vi "TemperatureToResistance.vi"(1 "Temperature / C":dbl=25.0, 2 "Bridge settings":T1) -> (0 "Resistance / Ohms":dbl=6247.958889803574 format="%0.2f")   [LabVIEW 2015]
uses:
  controls/BridgeSettings.ctl
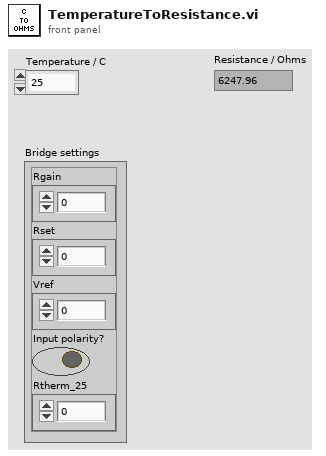
[diagram p1: front panel]
types:
  T1 = typedef "BridgeSettings.ctl" = cluster{"Rgain":dbl, "Rset":dbl, "Vref":dbl, "Input polarity?":bool, "Rtherm_25":dbl}
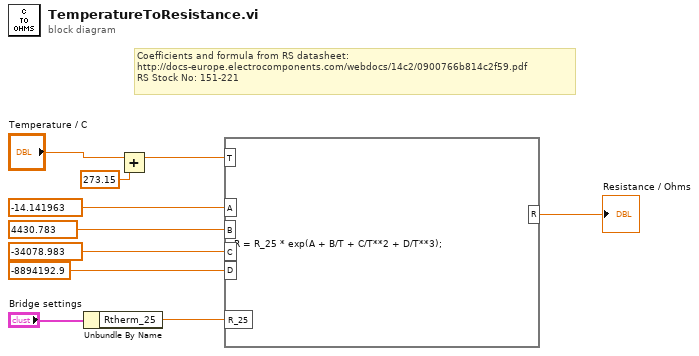
[diagram p0: block diagram]
diagram:
  # "Coefficients and formula from RS datasheet:\nhttp://docs-europe.electrocomponents.com/webdocs/14c2/0900766b814c2f59.pdf\nRS Stock No: 151-221"
  n1 = Unbundle By Name("Bridge settings") -> ("Rtherm_25"=w1:dbl)
  n2 = Add(x="Temperature / C", y=273.15) -> (x+y=w5:dbl)
  n3 = formula code="R = R_25 * exp(A + B/T + C/T**2 + D/T**3);"("A"=-14.141963, "B"=4430.783, "C"=-34078.983, "T"=w5, "D"=-8894192.9 ("input variable"), "R_25"=w1) -> ("R"=→"Resistance / Ohms":dbl)
